vi "Do.vi"(8 "error in (no error)":errorcluster, 10 "Actor in":refnum<class "Actor.lvclass">, 11 "Change Speaker Switch":refnum<class "Change Speaker Switch MSG.lvclass">) -> (0 "error out":errorcluster, 2 "Actor out":refnum<class "Actor.lvclass">)   [LabVIEW 2014, in "ePAS Library.lvlib" / "Change Speaker Switch MSG.lvclass"]
doc: "(<B>Filename</B>: Actor Framework.lvlib:Message.lvclass:Do.vi)\n\nDefines what a message does when it is received by an actor. Generally, a message instructs an actor to invoke one of its methods. By default, this method does nothing. A child class must override it to define behavior. Create a child class by using the Actor Framework Message Maker dialog box."
uses:
  Change Speaker Switch MSG.lvclass
  <vilib>/ActorFramework/Actor/Actor.lvclass
  Controller/Messages/Update Switch State MSG/Update Switch MSG.lvclass/Update Switch MSG.ctl
  Instr Actor.lvclass
  PAS/Commands/Change Speaker State/Change Speaker State.lvclass
  Controller/Messages/Update CVT/Update CVT Data.lvclass
  Controller/Messages/Update CVT/Update CVT Data.lvclass/Update CVT Data.ctl
  Controller/Messages/Update CVT/Write tag.vi
  Controller/Messages/Update CVT/Write Data.vi
  Controller/Messages/Update CVT/Write Group.vi
  Controller/Messages/Update Switch State MSG/Read Val.vi
  reusable/Command/Command.lvclass
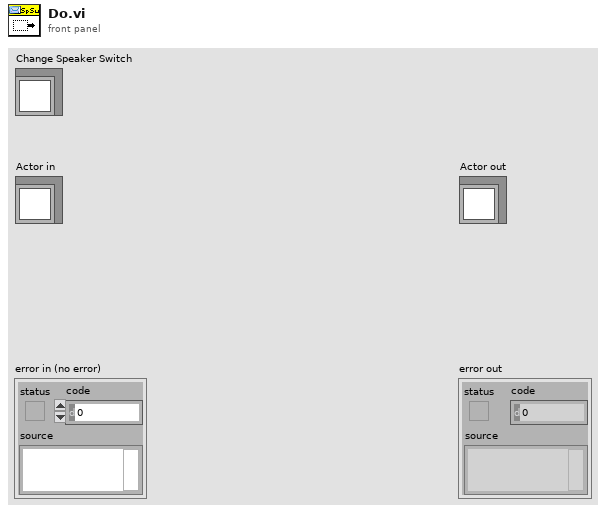
[diagram p1: front panel]
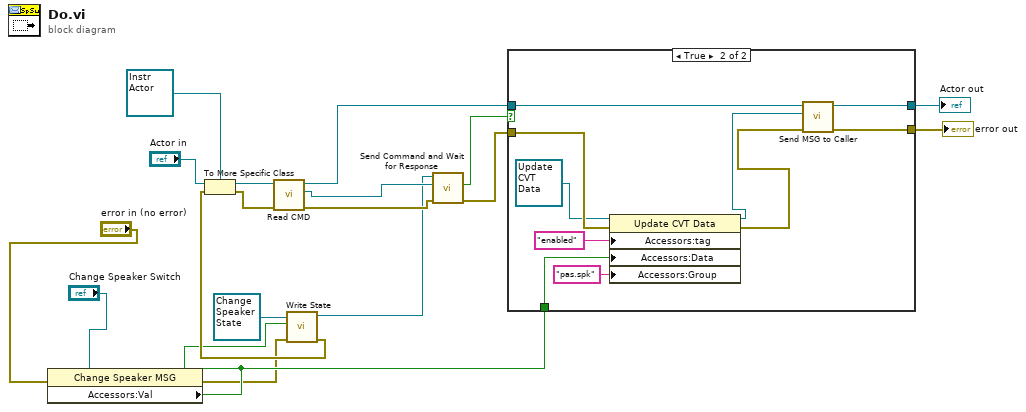
[diagram p0: block diagram]
diagram:
  n1 = property class="Change Speaker MSG"(reference="Change Speaker Switch", error in="error in (no error)") -> (error out=w1:errorcluster, "Accessors:Val"=w3:bool)  [unwired: 1 out]
  n2 = call "Write State.vi"("error in (no error)"=w1, "State"=w3, "Change Speaker State in"=refnum<class "Change Speaker State.lvclass"> refnum ("Change Speaker State.lvclass")) -> ("error out"=w13:errorcluster, "Change Speaker State out"=w10:refnum<class "Change Speaker State.lvclass">)  [unwired: 7 in]
  n3 = To More Specific Class(target class=refnum<class "Instr Actor.lvclass"> refnum ("Instrument Lib:Instr"), reference="Actor in", error in=w13) -> (specific class reference=w16:refnum<class "Instr Actor.lvclass">, error out=w15:errorcluster)
  n4 = call "Read CMD.vi"("error in (no error)"=w15, "Instr Actor in"=w16) -> ("error out"=w12:errorcluster, "CMD"=w11:refnum<queue>, "Instr Actor out"=w8:refnum<class "Instr Actor.lvclass">)  [unwired: 7 in]
  n5 = call "Send Command and Wait for Response.vi"("error in"=w12, "cmd queue"=w11, "CMD in"=w10) -> ("error out"=w6:errorcluster, "cmd good?"=w9:bool)  [unwired: 6 in, 1 out]
  n6 = case shown="True" w9 {
    tunnel: w3 -> [_ w26]
    tunnel: w8 -> [w20 w30]
    tunnel: [w20 w29] -> w7
    tunnel: w6 -> [w19 w24]
    tunnel: [w19 w28] -> w5
    frame False {
    }
    frame True {
      n7 = property class="Update CVT Data"(reference=refnum<class "Update CVT Data.lvclass"> refnum ("Controller.lvlib:Update CVT Data"), error in=w24, "Accessors:tag"="enabled" ("Key"), "Accessors:Data"=w26, "Accessors:Group"="pas.spk" ("Group")) -> (reference out=w25:refnum<class "Update CVT Data.lvclass">, error out=w23:errorcluster)
      n8 = call "Send MSG to Caller.vi"("error in"=w23, "Message"=w25, "Instr in"=w30) -> ("error out"=w28:errorcluster, "Instr out"=w29:refnum<class "Instr Actor.lvclass">)  [unwired: 7 in]
    }
  }
  "error out" <- w5
  "Actor out" <- w7
